vi "Integer Check Rows.vi"(11 "Sudoku Int":u8[][](array[numeric])) -> (3 "Is Ok":bool)   [LabVIEW 2015, in "Sudoku Library.lvlib"]
doc: "Created IvanLis by LabVIEW Portal\nProfile: http://labviewportal.org/memberlist.php?mode=viewprofile&u=987\neMail: IvanLisanov@gMail.com\nTelegram: https://t.me/IvanLis"
uses:
  Sudoku Library.lvlib
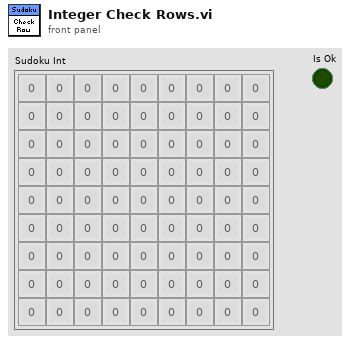
[diagram p1: front panel]
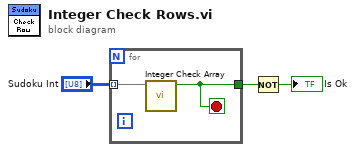
[diagram p0: block diagram]
diagram:
  n1 = for {
    tunnel: "Sudoku Int" -> [w5] mode=indexing
    tunnel: [w4] -> w2
    stop <- w4 stop-if-true
    n2 = call "Integer Check Array.vi"("Array"=w5) -> ("Error"=w4:bool)  [unwired: 10 in]
  }
  n3 = Not(x=w2) -> (.not. x?=→"Is Ok":bool)
